vi "Read Absolute Brushless Counter.vi"(8 "error in (no error)":errorcluster, 11 "VISA resource name":refnum<visa-resource-name>) -> (0 "error out":errorcluster, 2 "Encoder Speed (RPM)":i32, 3 "VISA resource name out":refnum<visa-resource-name>)   [LabVIEW 2012, in "Roboteq.lvlib"]
uses:
  Roboteq.lvlib
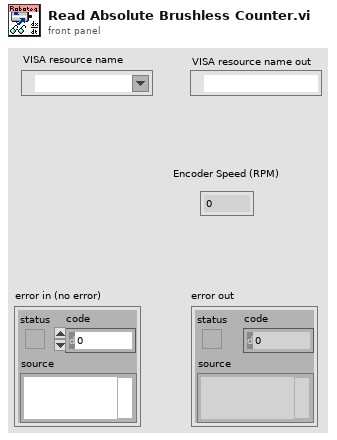
[diagram p1: front panel]
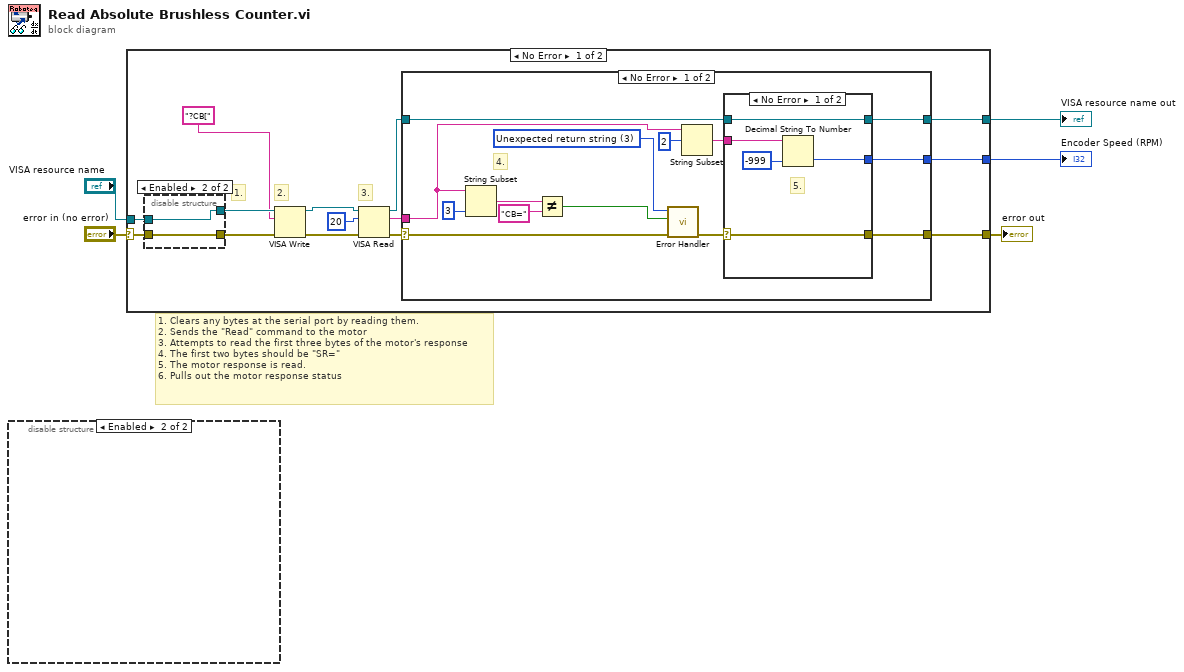
[diagram p0: block diagram]
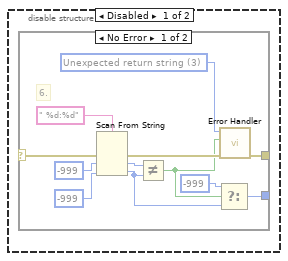
[diagram p2: hidden frame]
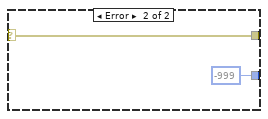
[diagram p3: hidden frame]
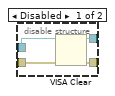
[diagram p4: hidden frame]
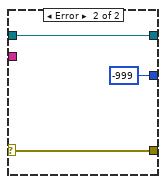
[diagram p5: hidden frame]
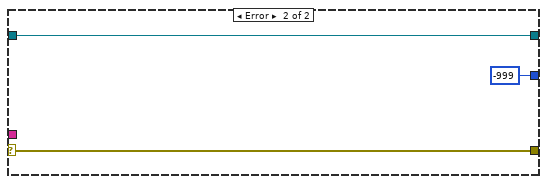
[diagram p6: hidden frame]
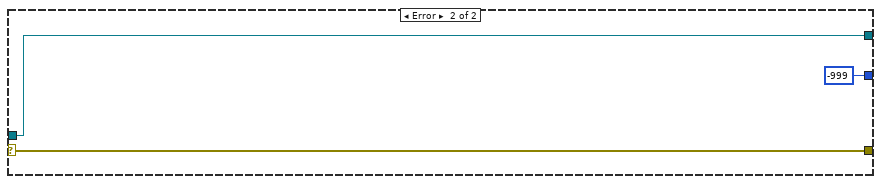
[diagram p7: hidden frame]
diagram:
  # "1. Clears any bytes at the serial port by reading them.\n2. Sends the \"Read\" command to the motor\n3. Attempts to read the first three bytes of the motor's response\n4. The first two bytes should be \"SR=\"\n5. The motor response is read.\n6. Pulls out the motor response status"
  n1 = disable-structure shown="Enabled" {
    frame Disabled {
      n2 = case shown="No Error" {
        selector: _ -> [w15 w18]
        tunnel: [w13 w18] -> _
        tunnel: [w10 -999 ("main battery\nvoltage (V)")] -> _
        frame No Error {
          w11 = u16 3 items=["Scan timeout"=1, "Invalid motor checksum"=2, "Unexpected return string"=3, "Invalid address range"=4] ("Error type")
          # "6."
          n3 = Scan From String(format string=" %d:%d", error in=w15, default 1=-999 ("default value 1"), default 2=-999 ("default value 1")) -> (error out=w12:errorcluster, output 1=w9:i32, output 2=w6:i32)  [unwired: 2 in, 2 out]
          n4 = Not Equal?(x=w9, y=w6) -> (x != y?=w7:bool)
          n5 = Select(t=-999 ("default value 1"), s=w7, f=w6) -> (s? t:f=w10:i32)
          n6 = call "Error Handler.vi"("error in (no error)"=w12, "Error? (no error)"=w7, "Error type"=w11) -> ("error out"=w13:errorcluster)  [unwired: 8 in]
        }
        frame Error {
        }
      }
    }
    frame Enabled {
    }
  }
  n7 = case shown="No Error" "error in (no error)" {
    selector: "error in (no error)" -> [w23 w67]
    tunnel: [w26 w67] -> w4
    tunnel: [w27 -999 ("main battery\nvoltage (V)")] -> w1
    tunnel: "VISA resource name" -> [w24 w65]
    tunnel: [w25 w65] -> w2
    frame No Error {
      # "3."
      # "2."
      # "1."
      n8 = disable-structure shown="Enabled" {
        disable-tunnel: w24 -> [w37 w38]
        disable-tunnel: w23 -> [w36 w39]
        disable-tunnel: [w35 w38] -> w22
        disable-tunnel: [w34 w39] -> w21
        frame Disabled {
          n9 = VISA Clear(VISA resource name=w37, error in (no error)=w36) -> (VISA resource name out=w35:refnum<visa-resource-name>, error out=w34:errorcluster)
        }
        frame Enabled {
        }
      }
      n10 = VISA Write(VISA resource name=w22, write buffer="?CB[" ("string"), error in (no error)=w21) -> (VISA resource name out=w32:refnum<visa-resource-name>, error out=w31:errorcluster)  [unwired: 1 out]
      n11 = VISA Read(VISA resource name=w32, byte count=u32 20, error in (no error)=w31) -> (VISA resource name out=w29:refnum<visa-resource-name>, read buffer=w28:string, error out=w30:errorcluster)  [unwired: 1 out]
      n12 = case shown="No Error" w30 {
        selector: w30 -> [w49 w64]
        tunnel: w28 -> [w42 _]
        tunnel: [w51 w64] -> w26
        tunnel: w29 -> [w53 w63]
        tunnel: [w52 w63] -> w25
        tunnel: [w45 -999 ("main battery\nvoltage (V)")] -> w27
        frame No Error {
          w46 = u16 3 items=["Scan timeout"=1, "Invalid motor checksum"=2, "Unexpected return string"=3, "Invalid address range"=4] ("Error type")
          # "4."
          n13 = String Subset(string=w42, length (rest)=3 ("length (rest)")) -> (substring=w41:string)  [unwired: 1 in]
          n14 = Not Equal?(x=w41, y="CB=" ("string")) -> (x != y?=w48:bool)
          n15 = call "Error Handler.vi"("error in (no error)"=w49, "Error? (no error)"=w48, "Error type"=w46) -> ("error out"=w50:errorcluster)  [unwired: 8 in]
          n16 = String Subset(string=w42, offset (0)=2 ("length (rest)")) -> (substring=w40:string)  [unwired: 1 in]
          n17 = case shown="No Error" w50 {
            selector: w50 -> [w54 w60]
            tunnel: w53 -> [w58 w61]
            tunnel: [w58 w61] -> w52
            tunnel: [w54 w60] -> w51
            tunnel: [w55 -999 ("main battery\nvoltage (V)")] -> w45
            tunnel: w40 -> [w57 _]
            frame No Error {
              # "5."
              n18 = Decimal String To Number(string=w57, default (0L)=-999 ("default (0 I32)")) -> (number=w55:i32)  [unwired: 1 in, 1 out]
            }
            frame Error {
            }
          }
        }
        frame Error {
        }
      }
    }
    frame Error {
    }
  }
  "VISA resource name out" <- w2
  "error out" <- w4
  "Encoder Speed (RPM)" <- w1
